vi "Update Messages.vi"(8 "error in (no error)":errorcluster, 10 "Messages":refnum<class "Message.lvclass">[](array[class]), 11 "Minor Frame in":refnum<class "Minor Frame.lvclass">) -> (0 "error out":errorcluster, 3 "Minor Frame out":refnum<class "Minor Frame.lvclass">)   [LabVIEW 2020, in "BCI-1553 API.lvlib" / "Minor Frame.lvclass"]
doc: "Adds or updates messages in the minor frame."
uses:
  Minor Frame.lvclass
  Message/Message.lvclass
  Minor Frame.lvclass/Minor Frame.ctl
  Dependencies/Registry/Registry.lvclass/Registry.ctl
  Dependencies/Registry/Add Entry.vi
  Dependencies/Registry/Registry.lvclass
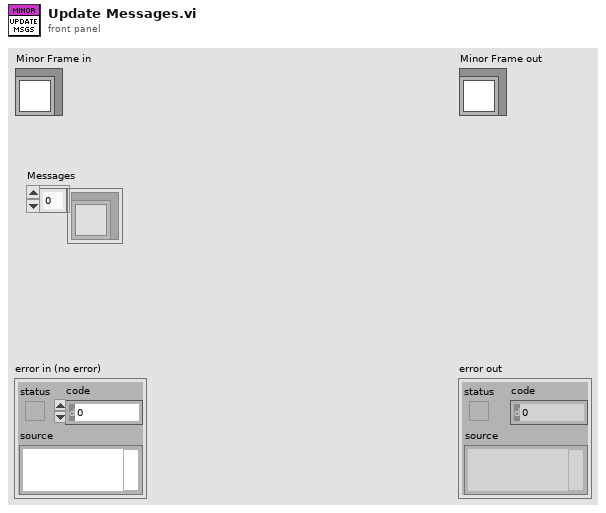
[diagram p1: front panel]
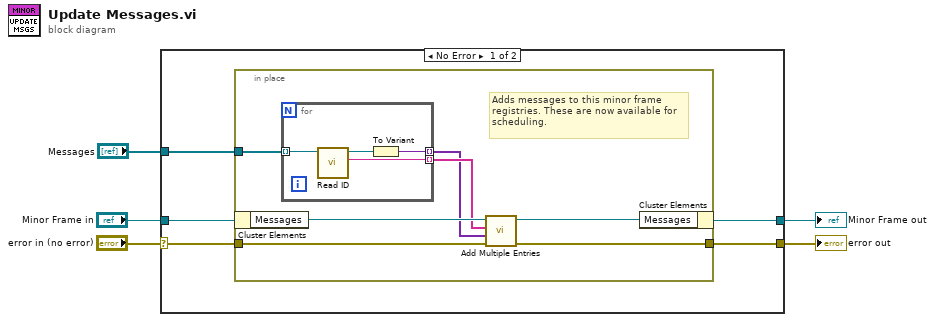
[diagram p0: block diagram]
diagram:
  n1 = case shown="No Error" "error in (no error)" {
    selector: "error in (no error)" -> [w7 w23]
    tunnel: [w8 w23] -> w3
    tunnel: [w9 w22] -> w2
    tunnel: "Minor Frame in" -> [w10 w22]
    tunnel: "Messages" -> [w6 _]
    frame No Error {
      n2 = in-place {
        in-place-border: [w15] -> w8
        in-place-border: w7 -> [w14]
        in-place-border: w6 -> [w13]
        # "Adds messages to this minor frame\nregistries. These are now available for\nscheduling."
        n3 = in-place-cluster #1(w10) -> ("Messages"=w17:refnum<class "Registry.lvclass">)
        n4 = for {
          tunnel: w13 -> [w20] mode=indexing
          tunnel: [w19] -> w12 mode=indexing
          tunnel: [w21] -> w11 mode=indexing
          n5 = call-dynamic "Read ID.vi"("Message in"=w20) -> ("ID"=w19:string, "Message out"=w18:refnum<class "Message.lvclass">)  [unwired: 8 in, 1 out]
          n6 = To Variant(anything=w18) -> (Variant=w21:variant)
        }
        n7 = call "Add Multiple Entries.vi"("error in (no error)"=w14, "Values"=w11, "Keys"=w12, "Registry in"=w17) -> ("error out"=w15:errorcluster, "Registry out"=w16:refnum<class "Registry.lvclass">)  [unwired: 5 in, 1 out]
        n8 = in-place-cluster #1("Messages"=w16) -> (w9:refnum<class "Minor Frame.lvclass">)
      }
    }
    frame Error {
    }
  }
  "error out" <- w3
  "Minor Frame out" <- w2
